vi "Write Operation.vi"(0 "I2C in":refnum<class "I2C.lvclass">, 11 "Error In":errorcluster) -> (4 "I2C out":refnum<class "I2C.lvclass">, 6 "Digial Waveform Data":digitalwaveform(waveform)={"t0"=timestamp(0 s since 1904-01-01), "dt"=1.0, "Y"={"transitions"=[], "data"=[]}}, 15 "Error Out":errorcluster)   [LabVIEW 2020, in "I2C Controller.lvlib" / "I2C.lvclass"]
uses:
  I2C.lvclass
  I2C.lvclass/I2C.ctl
panel:
  out "Digital Waveform Graph":digitalwaveform(graph)
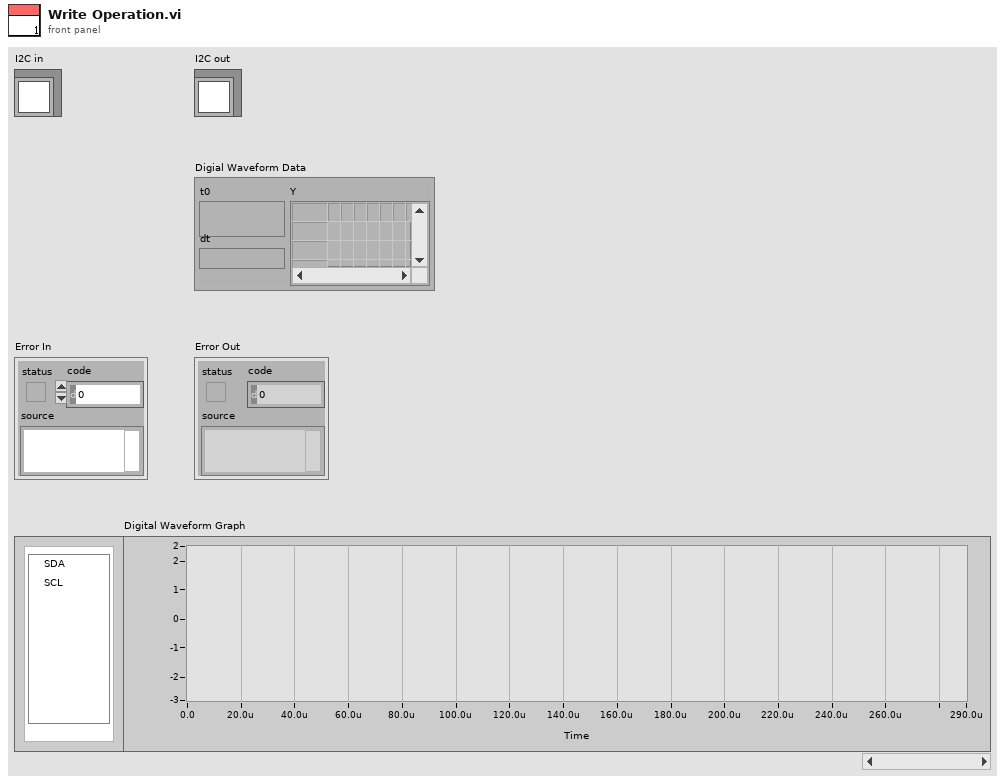
[diagram p1: front panel]
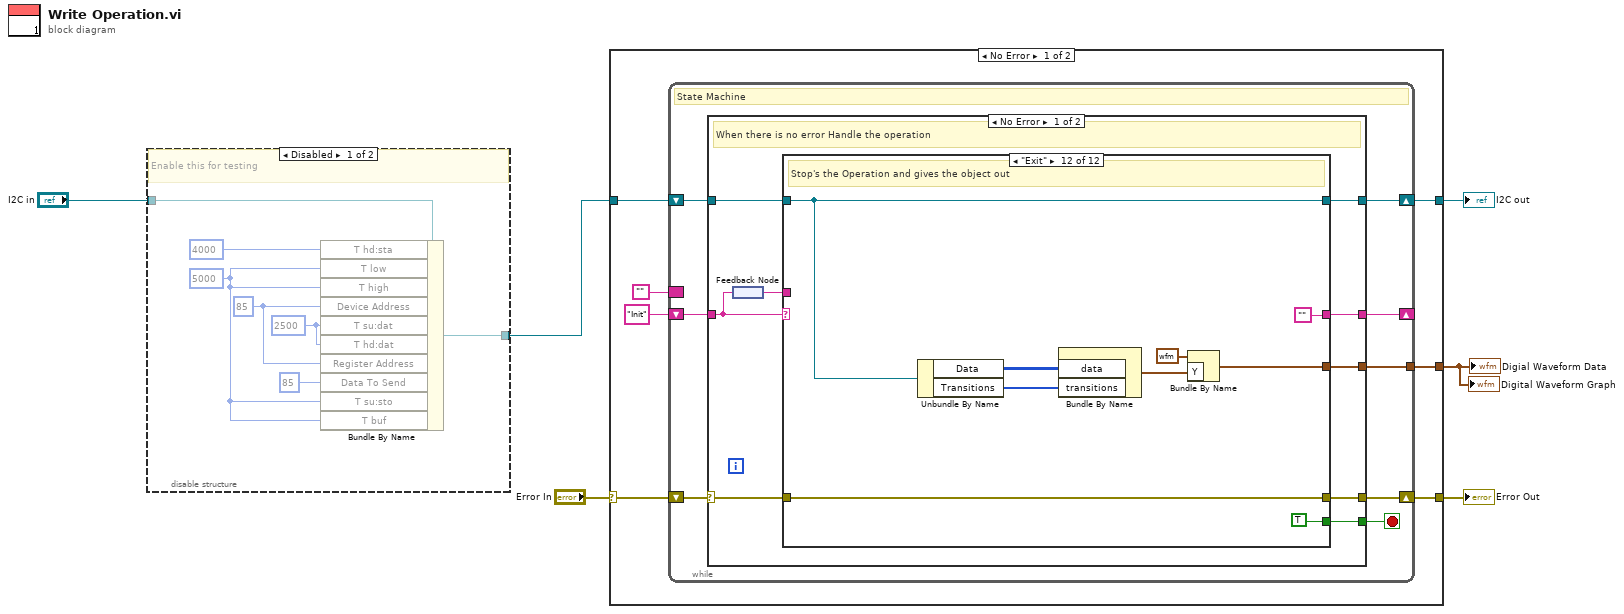
[diagram p0: block diagram]
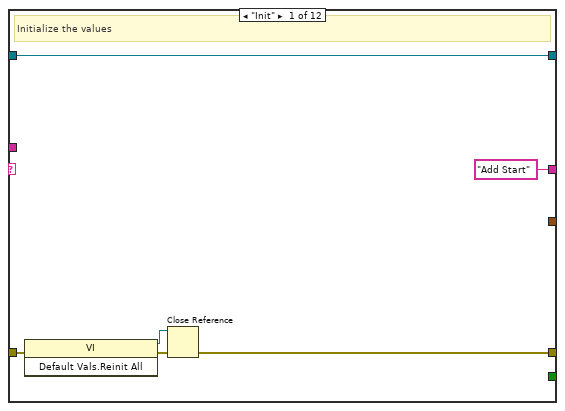
[diagram p3: hidden frame]
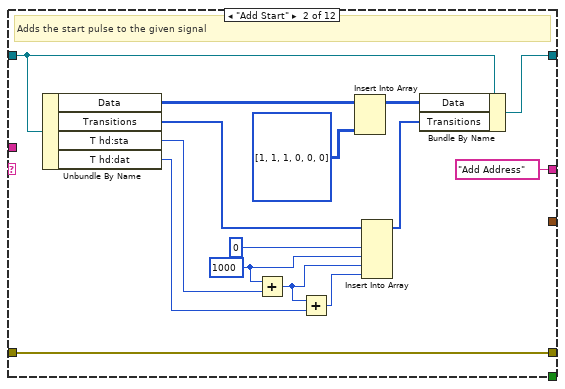
[diagram p4: hidden frame]
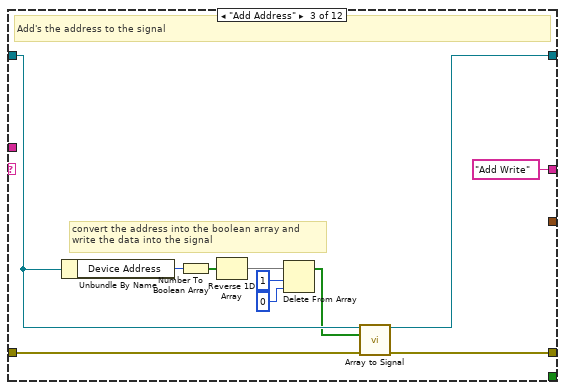
[diagram p5: hidden frame]
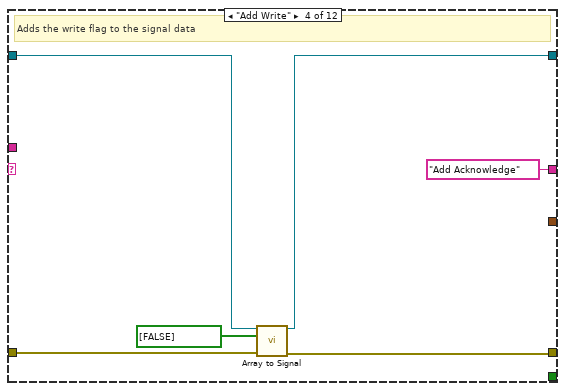
[diagram p6: hidden frame]
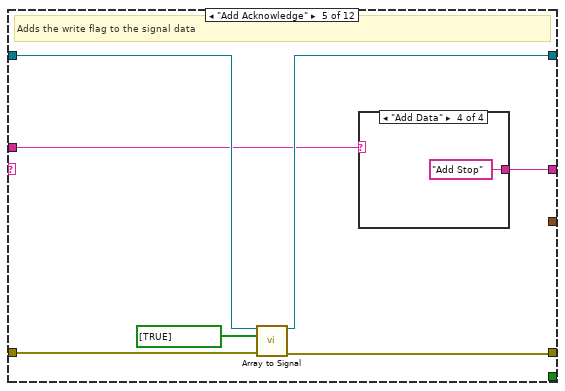
[diagram p7: hidden frame]
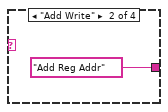
[diagram p9: hidden frame]
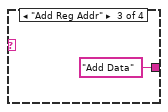
[diagram p10: hidden frame]
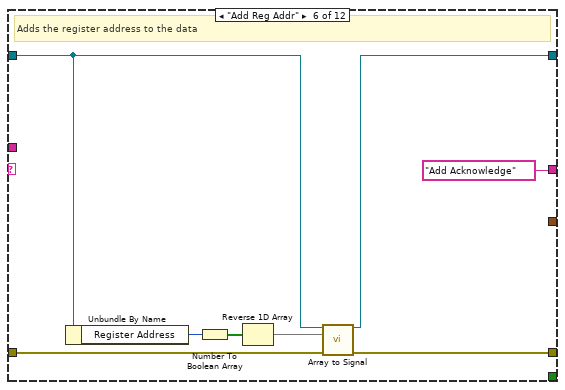
[diagram p11: hidden frame]
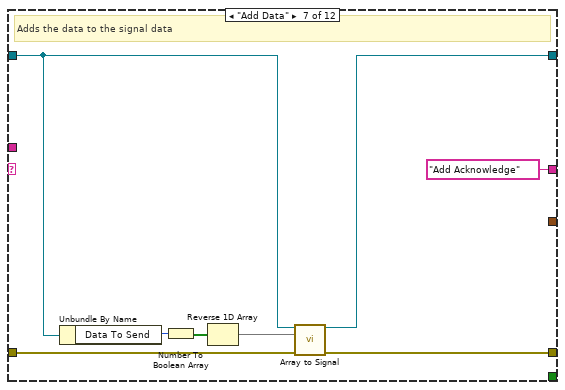
[diagram p12: hidden frame]
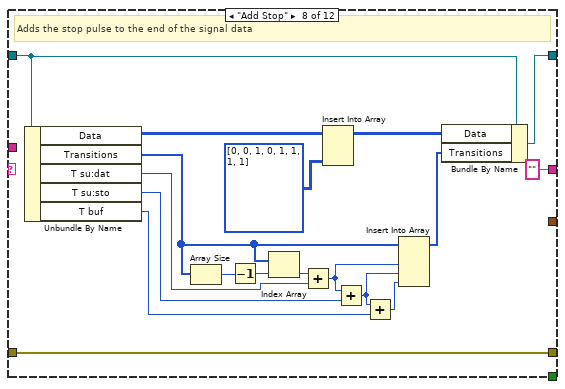
[diagram p13: hidden frame]
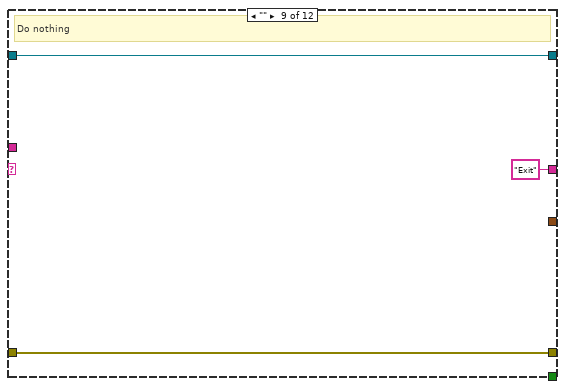
[diagram p14: hidden frame]
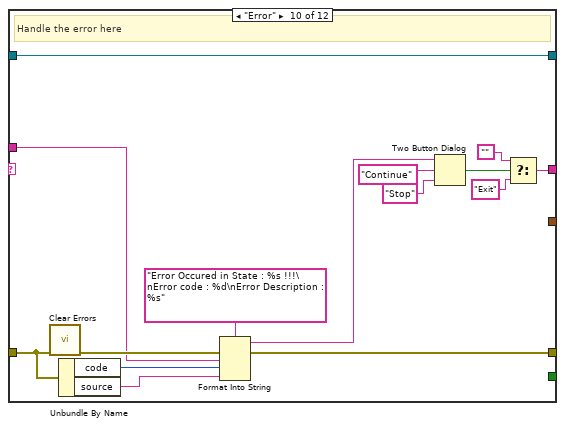
[diagram p15: hidden frame]
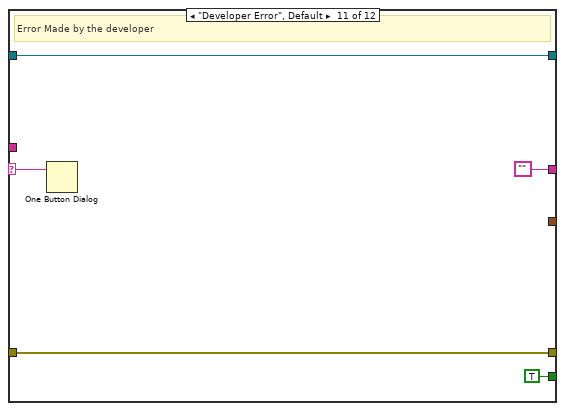
[diagram p16: hidden frame]
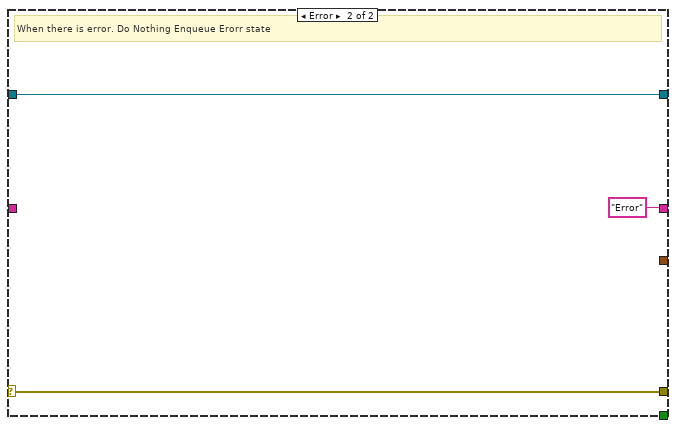
[diagram p17: hidden frame]
diagram:
  n1 = disable-structure shown="Disabled" {
    disable-tunnel: "I2C in" -> [w13 w14]
    disable-tunnel: [w12 w14] -> w2
    frame Disabled {
      w10 = u32 2500 ("Timings.T su:dat")
      w9 = u8 85 ("Device Address")
      w7 = u32 5000 ("Timings.T low")
      # "Enable this for testing"
      n2 = Bundle By Name(cluster=w13, "T hd:sta"=u32 4000 ("Timings.T hd:sta"), "T low"=w7, "T high"=w7, "Device Address"=w9, "T su:dat"=w10, "T hd:dat"=w10, "Register Address"=w9, "Data To Send"=u8 85 ("Data"), "T su:sto"=w7, "T buf"=w7) -> (w12:refnum<class "I2C.lvclass">)
    }
    frame Enabled {
    }
  }
  n3 = case shown="No Error" "Error In" {
    selector: "Error In" -> [w19 w157]
    tunnel: [w18 w157] -> w5
    tunnel: [w16 w156] -> w3
    tunnel: w2 -> [w17 w156]
    tunnel: [w15 _] -> w1
    frame No Error {
      n4 = while {
        shift-right: [w28] -> w18
        shift-left: w19 -> [w29]
        shift-right: [w27] -> _
        shift-left: "Init" -> [w26]
        border: "" -> [_]
        shift-right: [w23] -> w16
        shift-left: w17 -> [w24]
        tunnel: [w22] -> w15
        stop <- w25 stop-if-true
        # "State Machine"
        n5 = case shown="No Error" w29 {
          selector: w29 -> [w38 w155]
          tunnel: [w37 w155] -> w28
          tunnel: [w36 "Error"] -> w27
          tunnel: w26 -> [w34 _]
          tunnel: [w35 _] -> w25
          tunnel: w24 -> [w32 w153]
          tunnel: [w31 w153] -> w23
          tunnel: [w30 _] -> w22
          frame No Error {
            # "When there is no error Handle the operation"
            n6 = feedback #1() -> (w33:string)
            n7 = feedback-in #1(w34) -> ()
            n8 = case shown="\"Exit\"" w34 {
              selector: w34 -> [_ _ _ _ _ _ _ _ _ _ w141 _]
              tunnel: [w41 w59 w63 w75 w82 w93 w101 w120 w123 w136 w143 w150] -> w37
              tunnel: w38 -> [w44 w59 w70 w76 w83 w94 w102 w120 w123 w137 w143 w150]
              tunnel: ["Add Start" "Add Address" "Add Write" "Add Acknowledge" w77 "Add Acknowledge" "Add Acknowledge" "" "Exit" w127 "" ""] -> w36
              tunnel: [_ _ _ _ _ _ _ _ _ _ TRUE TRUE] -> w35
              tunnel: w33 -> [_ _ _ _ w78 _ _ _ _ w135 _ _]
              tunnel: [w39 w57 w62 w74 w81 w92 w100 w119 w122 w124 w140 w149] -> w31
              tunnel: w32 -> [w39 w58 w61 w73 w80 w91 w99 w118 w122 w124 w140 w149]
              tunnel: [_ _ _ _ _ _ _ _ _ _ _ w144] -> w30
              frame "Init" {
                # "Initialize the values"
                n9 = invoke class="VI" method="Default Vals.Reinit All"(error in=w44) -> (reference out=w40:refnum<vi>, error out=w42:errorcluster)  [unwired: 2 in, 1 out]
                n10 = Close Reference(reference=w40, error in (no error)=w42) -> (error out=w41:errorcluster)
              }
              frame "Add Start" {
                w48 = u32 1000 ("new element/subarray")
                # "Adds the start pulse to the given signal"
                n11 = Unbundle By Name(w58) -> ("Data"=w56:u8[][], "Transitions"=w55:u32[], "T hd:sta"=w51:u32, "T hd:dat"=w46:u32)
                n12 = Add(x=w48, y=w51) -> (x+y=w47:u32)
                n13 = Add(x=w47, y=w46) -> (x+y=w45:u32)
                n14 = Insert Into Array(array=w56, new element=u8[][] [[1, 1], [1, 0], [0, 0]] ("Data")) -> (w53:u8[][])  [unwired: 2 in]
                n15 = Insert Into Array(array=w55, new element #1=u32 0 ("new element/subarray"), new element #2=w48, new element #3=w47, new element #4=w45) -> (w54:u32[])  [unwired: 1 in]
                n16 = Bundle By Name(cluster=w58, "Data"=w53, "Transitions"=w54) -> (w57:refnum<class "I2C.lvclass">)
              }
              frame "Add Address" {
                # "convert the address into the boolean array and\nwrite the data into the signal"
                # "Add's the address to the signal"
                n17 = Unbundle By Name(w61) -> ("Device Address"=w68:u8)
                n18 = Number To Boolean Array(number=w68) -> (Boolean array=w67:bool[])
                n19 = Reverse 1D Array(array=w67) -> (reversed array=w66:bool[])
                n20 = Delete From Array(array=w66, length=1, index=0) -> (array with subset deleted=w60:bool[])  [unwired: 1 out]
                n21 = call "Array to Signal.vi"("I2C in"=w61, "Data Array"=w60, "Error In"=w70) -> ("I2C out"=w62:refnum<class "I2C.lvclass">, "Error Out"=w63:errorcluster)  [unwired: 11 in]
              }
              frame "Add Write" {
                # "Adds the write flag to the signal data"
                n22 = call "Array to Signal.vi"("I2C in"=w73, "Data Array"=bool[] [FALSE], "Error In"=w76) -> ("I2C out"=w74:refnum<class "I2C.lvclass">, "Error Out"=w75:errorcluster)  [unwired: 11 in]
              }
              frame "Add Acknowledge" {
                # "Adds the write flag to the signal data"
                n23 = call "Array to Signal.vi"("I2C in"=w80, "Data Array"=bool[] [TRUE], "Error In"=w83) -> ("I2C out"=w81:refnum<class "I2C.lvclass">, "Error Out"=w82:errorcluster)  [unwired: 11 in]
                n24 = case shown="\"Add Data\"" w78 {
                  tunnel: [_ "Add Reg Addr" "Add Data" "Add Stop"] -> w77
                  frame Default {
                  }
                  frame "Add Write" {
                  }
                  frame "Add Reg Addr" {
                  }
                  frame "Add Data" {
                  }
                }
              }
              frame "Add Reg Addr" {
                # "Adds the register address to the data"
                n25 = Unbundle By Name(w91) -> ("Register Address"=w90:u8)
                n26 = Number To Boolean Array(number=w90) -> (Boolean array=w89:bool[])
                n27 = Reverse 1D Array(array=w89) -> (reversed array=w88:bool[])
                n28 = call "Array to Signal.vi"("I2C in"=w91, "Data Array"=w88, "Error In"=w94) -> ("I2C out"=w92:refnum<class "I2C.lvclass">, "Error Out"=w93:errorcluster)  [unwired: 11 in]
              }
              frame "Add Data" {
                # "Adds the data to the signal data"
                n29 = Unbundle By Name(w99) -> ("Data To Send"=w98:u8)
                n30 = Number To Boolean Array(number=w98) -> (Boolean array=w97:bool[])
                n31 = Reverse 1D Array(array=w97) -> (reversed array=w96:bool[])
                n32 = call "Array to Signal.vi"("I2C in"=w99, "Data Array"=w96, "Error In"=w102) -> ("I2C out"=w100:refnum<class "I2C.lvclass">, "Error Out"=w101:errorcluster)  [unwired: 11 in]
              }
              frame "Add Stop" {
                # "Adds the stop pulse to the end of the signal data"
                n33 = Unbundle By Name(w118) -> ("Data"=w117:u8[][], "Transitions"=w110:u32[], "T su:dat"=w108:u32, "T su:sto"=w103:u32, "T buf"=w104:u32)
                n34 = Array Size(array=w110) -> (size(s)=w112:i32)
                n35 = Decrement(x=w112) -> (x-1=w111:i32)
                n36 = Index Array(array=w110, index=w111) -> (element=w109:u32)
                n37 = Add(x=w109, y=w108) -> (x+y=w107:u32)
                n38 = Insert Into Array(array=w117, new element=u8[][] [[0, 0], [1, 0], [1, 1], [1, 1]] ("Data")) -> (w114:u8[][])  [unwired: 2 in]
                n39 = Add(x=w107, y=w103) -> (x+y=w106:u32)
                n40 = Add(x=w106, y=w104) -> (x+y=w105:u32)
                n41 = Insert Into Array(array=w110, new element #1=w107, new element #2=w106, new element #3=w105) -> (w115:u32[])  [unwired: 1 in]
                n42 = Bundle By Name(cluster=w118, "Data"=w114, "Transitions"=w115) -> (w119:refnum<class "I2C.lvclass">)
              }
              frame "" {
                # "Do nothing"
              }
              frame "Error" {
                # "Handle the error here"
                n43 = call <vilib>:"Clear Errors.vi"("error in (no error)"=w137) -> ("error out"=w138:errorcluster)  [unwired: 5 in, 1 out]
                n44 = Unbundle By Name(w137) -> ("code"=w134:i32, "source"=w133:string)
                n45 = Format Into String(format string="Error Occured in State : %s !!!\nError code : %d\nError Description : %s", error in=w138, w135, w134, w133) -> (resulting string=w131:string, error out=w136:errorcluster)  [unwired: 1 in]
                n46 = Two Button Dialog(message=w131, 1:"Stop" ("F button name (\"Cancel\")"), 2:"Continue" ("T button name (\"OK\")")) -> (T button?=w128:bool)
                n47 = Select(t="", s=w128, f="Exit") -> (s? t:f=w127:string)
              }
              frame "Developer Error", Default {
                # "Error Made by the developer"
                n48 = One Button Dialog(message=w141) -> ()  [unwired: 1 in, 1 out]
              }
              frame "Exit" {
                # "Stop's the Operation and gives the object out"
                n49 = Unbundle By Name(w149) -> ("Data"=w146:u8[][], "Transitions"=w145:u32[])
                n50 = Bundle By Name("data"=w146, "transitions"=w145) -> (w148:digitaldata)  [unwired: 1 in]
                n51 = Bundle By Name(cluster=digitalwaveform {"t0"=timestamp(0 s since 1904-01-01), "dt"=1e-09, "Y"={"transitions"=[], "data"=[]}} ("waveform"), "Y"=w148) -> (w144:digitalwaveform)
              }
            }
          }
          frame Error {
            # "When there is error. Do Nothing Enqueue Erorr state"
          }
        }
      }
    }
    frame Error {
    }
  }
  "Error Out" <- w5
  "I2C out" <- w3
  "Digital Waveform Graph" <- w1
  "Digial Waveform Data" <- w1
